vi "safe shoot error.vi"(1 "Can Shoot Safely?":bool, 2 "Menu":T1) -> (0 "Can Shoot Safely?":bool)   [LabVIEW 2013]
uses:
  typedefs/fg_typedef.ctl
panel:
  # "Has the robot met the prerequisites for shooting safely?"
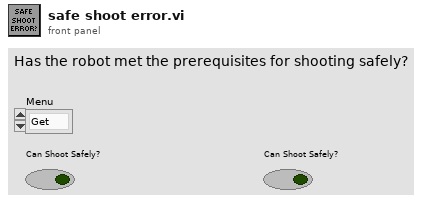
[diagram p1: front panel]
types:
  T1 = typedef "fg_typedef.ctl" = enum16{"Get", "Set"}
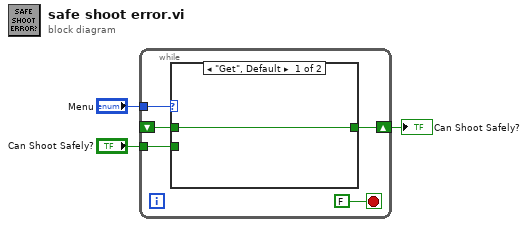
[diagram p0: block diagram]
diagram:
  n1 = while {
    tunnel: "Menu" -> [w8]
    tunnel: "Can Shoot Safely?" -> [w7]
    shift-right: [w6] -> w1
    shift-left: _ -> [w5]
    stop <- FALSE stop-if-true
    n2 = case shown="\"Get\", Default" w8 {
      tunnel: w7 -> [_ w10]
      tunnel: [w9 w10] -> w6
      tunnel: w5 -> [w9 _]
      frame "Get", Default {
      }
      frame "Set" {
      }
    }
  }
  "Can Shoot Safely?" <- w1
